vi "resave_camera_images.vi"() -> ()   [LabVIEW 2019]
uses:
  <vilib>/vision/NI_Vision_Development_Module.lvlib
panel:
  out "Processed Frames/s 8":dbl
  out "Processed Frames/s 7":dbl
  out "Processed Frames/s 6":dbl
  out "Processed Frames/s 5":dbl
  out "Processed Frames/s 4":dbl
  out "Processed Frames/s 3":dbl
  out "Processed Frames/s 2":dbl
  out "Processed Frames/s":dbl
  out "error out":errorcluster
  in  "Experiment Folder In":string="C:\\Data\\20200217_HeadTailContinuousGWN_test\\Data20200217_115033\\"
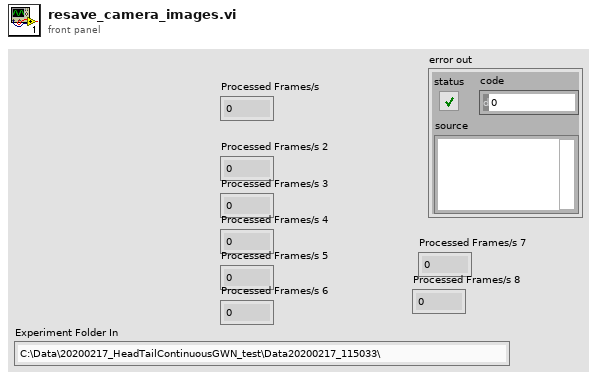
[diagram p1: front panel]
types:
  T1 = typedef "Image Type" = u32
  T2 = typedef "IMAQ Image.ctl" = refnum<image>
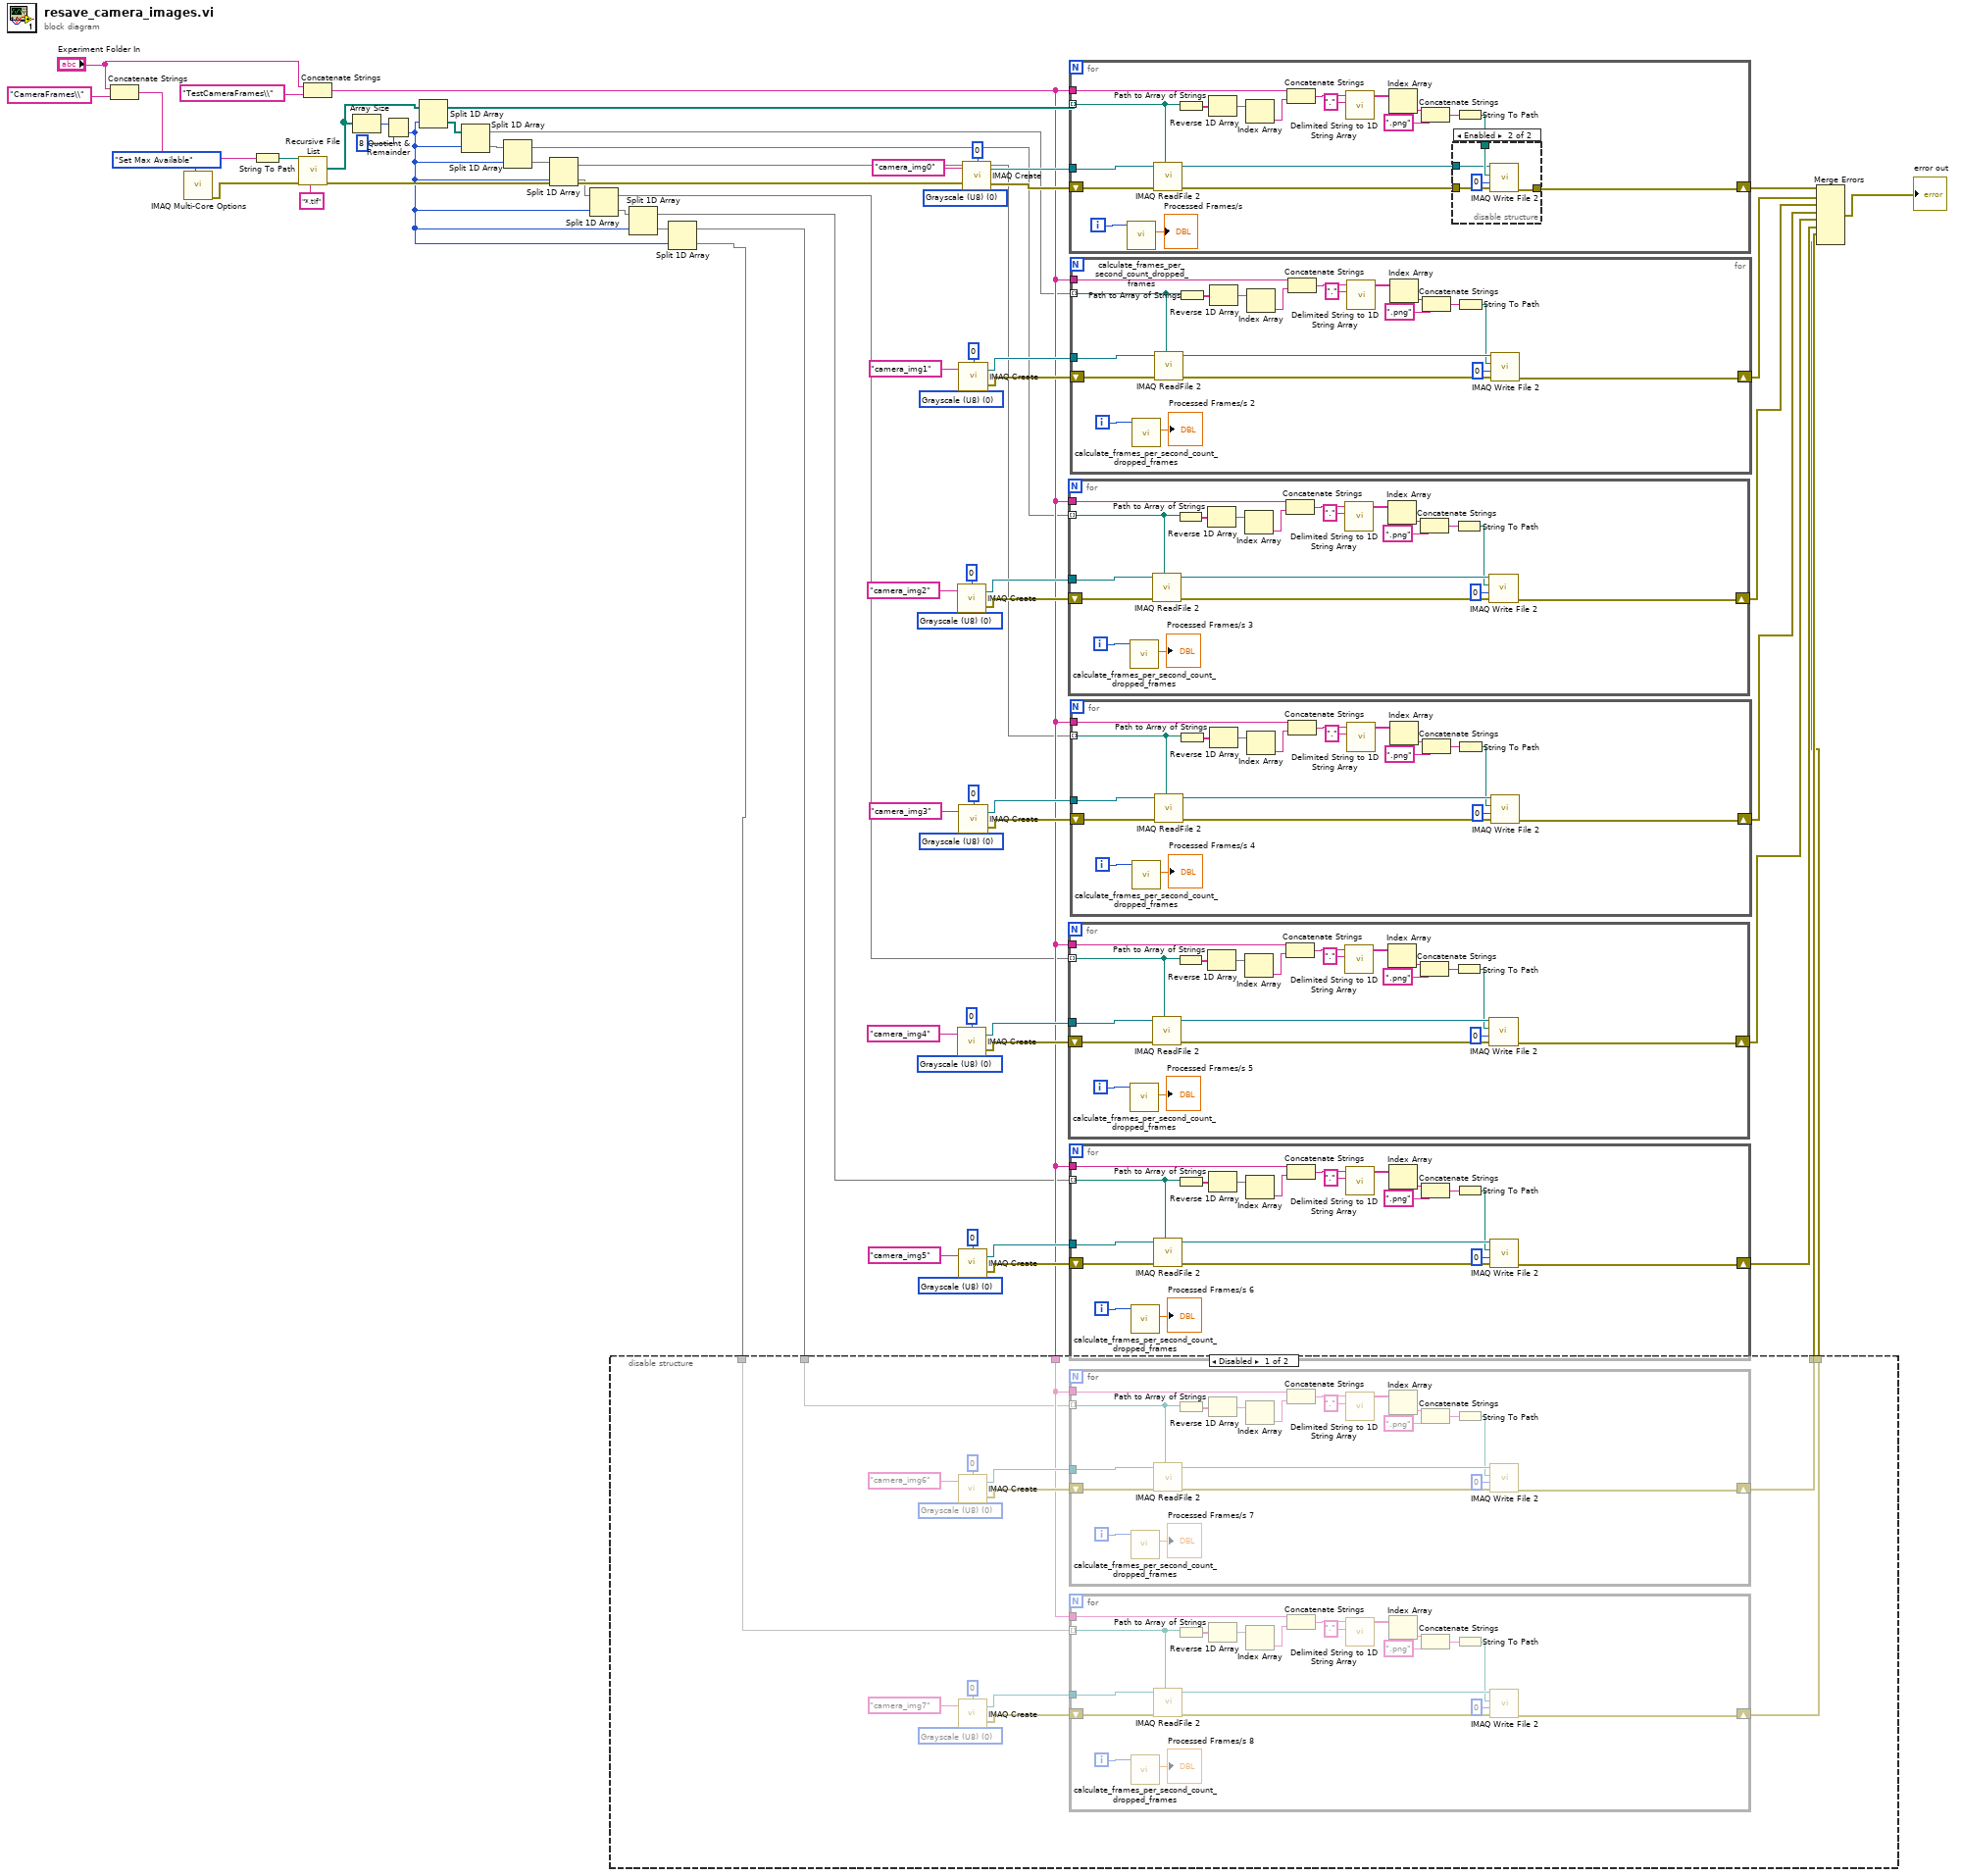
[diagram p0: block diagram]
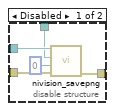
[diagram p3: hidden frame]
diagram:
  w24 = T1 0 items=["Grayscale (U8)", "Grayscale (I16)", "Grayscale (SGL)", "Complex (CSG)", "RGB (U32)", "HSL (U32)", "RGB (U64)", "Grayscale (U16)"] ("Image Type")
  w29 = T1 0 items=["Grayscale (U8)", "Grayscale (I16)", "Grayscale (SGL)", "Complex (CSG)", "RGB (U32)", "HSL (U32)", "RGB (U64)", "Grayscale (U16)"] ("Image Type")
  w34 = T1 0 items=["Grayscale (U8)", "Grayscale (I16)", "Grayscale (SGL)", "Complex (CSG)", "RGB (U32)", "HSL (U32)", "RGB (U64)", "Grayscale (U16)"] ("Image Type")
  w39 = T1 0 items=["Grayscale (U8)", "Grayscale (I16)", "Grayscale (SGL)", "Complex (CSG)", "RGB (U32)", "HSL (U32)", "RGB (U64)", "Grayscale (U16)"] ("Image Type")
  w52 = T1 0 items=["Grayscale (U8)", "Grayscale (I16)", "Grayscale (SGL)", "Complex (CSG)", "RGB (U32)", "HSL (U32)", "RGB (U64)", "Grayscale (U16)"] ("Image Type")
  w61 = T1 0 items=["Grayscale (U8)", "Grayscale (I16)", "Grayscale (SGL)", "Complex (CSG)", "RGB (U32)", "HSL (U32)", "RGB (U64)", "Grayscale (U16)"] ("Image Type")
  n1 = Concatenate Strings("Experiment Folder In", "CameraFrames\\" ("string")) -> (w66:string)
  n2 = call "IMAQ Multi-Core Options"("Get/Set Number of Cores (Get)"=enum32{"Get", "Set", "Set Max Available"}."Set Max Available") -> ("error out"=w42:errorcluster)  [unwired: 9 in, 1 out]
  n3 = String To Path(string=w66) -> (path=w64:path)
  n4 = call <vilib>:"Recursive File List.vi"("pattern"="*.tif", "error in (no error)"=w42, "Folder Path"=w64) -> ("error out"=w58:errorcluster, "All Files in Dir"=w49:path[])  [unwired: 4 in, 3 out]
  n5 = Concatenate Strings("Experiment Folder In", "TestCameraFrames\\" ("string")) -> (w21:string)
  n6 = Array Size(array=w49) -> (size(s)=w48:i32)
  n7 = Quotient & Remainder(x=w48, y=8) -> (floor(x/y)=w2:i32)  [unwired: 1 out]
  n8 = Split 1D Array(array=w49, index=w2) -> (first subarray=w55:path[], second subarray=w14:path[])
  n9 = Split 1D Array(array=w14, index=w2) -> (first subarray=w13:path[], second subarray=w12:path[])
  n10 = Split 1D Array(array=w12, index=w2) -> (first subarray=w11:path[], second subarray=w10:path[])
  n11 = Split 1D Array(array=w10, index=w2) -> (first subarray=w9:path[], second subarray=w8:path[])
  n12 = Split 1D Array(array=w8, index=w2) -> (first subarray=w7:path[], second subarray=w6:path[])
  n13 = Split 1D Array(array=w6, index=w2) -> (first subarray=w5:path[], second subarray=w4:path[])
  n14 = Split 1D Array(array=w4, index=w2) -> (first subarray=w3:path[], second subarray=w1:path[])
  n15 = disable-structure shown="Disabled" {
    disable-tunnel: w21 -> [w72 _]
    disable-tunnel: [w71 _] -> w16
    disable-tunnel: [w70 _] -> w15
    disable-tunnel: w3 -> [w69 _]
    disable-tunnel: w1 -> [w68 _]
    frame Disabled {
      w75 = T1 0 items=["Grayscale (U8)", "Grayscale (I16)", "Grayscale (SGL)", "Complex (CSG)", "RGB (U32)", "HSL (U32)", "RGB (U64)", "Grayscale (U16)"] ("Image Type")
      w80 = T1 0 items=["Grayscale (U8)", "Grayscale (I16)", "Grayscale (SGL)", "Complex (CSG)", "RGB (U32)", "HSL (U32)", "RGB (U64)", "Grayscale (U16)"] ("Image Type")
      n16 = call "IMAQ Create"("Border Size"=0, "Image Name"="camera_img6", "Image Type"=w80) -> ("New Image"=w78:T2, "error out"=w79:errorcluster)  [unwired: 2 in]
      n17 = call "IMAQ Create"("Border Size"=0, "Image Name"="camera_img7", "Image Type"=w75) -> ("New Image"=w73:T2, "error out"=w74:errorcluster)  [unwired: 2 in]
      n18 = for {
        tunnel: w69 -> [w116] mode=indexing
        tunnel: w78 -> [w122]
        tunnel: w72 -> [w115]
        shift-right: [w112] -> w71
        shift-left: w79 -> [w121]
        i -> [w111]
        n19 = call "calculate_frames_per_second_count_dropped_frames.vi"("Buffer Number"=w111) -> ("Processed Frames/s"=→"Processed Frames/s 7":dbl)  [unwired: 8 in, 2 out]
        n20 = call "IMAQ ReadFile 2"("File Path"=w116, "error in (no error)"=w121, "Image"=w122) -> ("error out"=w120:errorcluster, "Image Out"=w119:T2)  [unwired: 4 in, 3 out]
        n21 = Path to Array of Strings(0:w116) -> (2:w118:string[])  [unwired: 1 out]
        n22 = Reverse 1D Array(array=w118) -> (reversed array=w117:string[])
        n23 = Index Array(array=w117) -> (element=w114:string)  [unwired: 1 in]
        n24 = Concatenate Strings(w115, w114) -> (w109:string)
        n25 = call <vilib>:"Delimited String to 1D String Array.vi"("delimiter"=".", "delimited string"=w109) -> ("string array"=w107:string[])  [unwired: 9 in]
        n26 = Index Array(array=w107) -> (element=w106:string)  [unwired: 1 in]
        n27 = Concatenate Strings(w106, ".png" ("string")) -> (w104:string)
        n28 = String To Path(string=w104) -> (path=w113:path)
        n29 = call-poly "IMAQ Write File 2"("error in (no error)"=w120, "Image Quality"=u32 0, "File Path"=w113, "Image"=w119) -> ("error out"=w112:errorcluster)  [unwired: 6 in, 1 out]
      }
      n30 = for {
        tunnel: w68 -> [w96] mode=indexing
        tunnel: w73 -> [w102]
        tunnel: w72 -> [w95]
        shift-right: [w92] -> w70
        shift-left: w74 -> [w101]
        i -> [w91]
        n31 = call "calculate_frames_per_second_count_dropped_frames.vi"("Buffer Number"=w91) -> ("Processed Frames/s"=→"Processed Frames/s 8":dbl)  [unwired: 8 in, 2 out]
        n32 = call "IMAQ ReadFile 2"("File Path"=w96, "error in (no error)"=w101, "Image"=w102) -> ("error out"=w100:errorcluster, "Image Out"=w99:T2)  [unwired: 4 in, 3 out]
        n33 = Path to Array of Strings(0:w96) -> (2:w98:string[])  [unwired: 1 out]
        n34 = Reverse 1D Array(array=w98) -> (reversed array=w97:string[])
        n35 = Index Array(array=w97) -> (element=w94:string)  [unwired: 1 in]
        n36 = Concatenate Strings(w95, w94) -> (w89:string)
        n37 = call <vilib>:"Delimited String to 1D String Array.vi"("delimiter"=".", "delimited string"=w89) -> ("string array"=w87:string[])  [unwired: 9 in]
        n38 = Index Array(array=w87) -> (element=w86:string)  [unwired: 1 in]
        n39 = Concatenate Strings(w86, ".png" ("string")) -> (w84:string)
        n40 = String To Path(string=w84) -> (path=w93:path)
        n41 = call-poly "IMAQ Write File 2"("error in (no error)"=w100, "Image Quality"=u32 0, "File Path"=w93, "Image"=w99) -> ("error out"=w92:errorcluster)  [unwired: 6 in, 1 out]
      }
    }
    frame Enabled {
    }
  }
  n42 = call "IMAQ Create"("Border Size"=0, "Image Name"="camera_img2", "Image Type"=w39) -> ("New Image"=w37:T2, "error out"=w38:errorcluster)  [unwired: 2 in]
  n43 = call "IMAQ Create"("Border Size"=0, "Image Name"="camera_img4", "Image Type"=w29) -> ("New Image"=w27:T2, "error out"=w28:errorcluster)  [unwired: 2 in]
  n44 = call "IMAQ Create"("Border Size"=0, "Image Name"="camera_img5", "Image Type"=w24) -> ("New Image"=w22:T2, "error out"=w23:errorcluster)  [unwired: 2 in]
  n45 = call "IMAQ Create"("Border Size"=0, "Image Name"="camera_img1", "Image Type"=w52) -> ("New Image"=w50:T2, "error out"=w51:errorcluster)  [unwired: 2 in]
  n46 = call "IMAQ Create"("Border Size"=0, "Image Name"="camera_img3", "Image Type"=w34) -> ("New Image"=w32:T2, "error out"=w33:errorcluster)  [unwired: 2 in]
  n47 = call "IMAQ Create"("Border Size"=0, "Image Name"="camera_img0", "Image Type"=w61, "error in (no error)"=w58) -> ("New Image"=w60:T2, "error out"=w59:errorcluster)  [unwired: 1 in]
  n48 = for {
    tunnel: w11 -> [w136] mode=indexing
    tunnel: w37 -> [w142]
    tunnel: w21 -> [w135]
    shift-right: [w132] -> w20
    shift-left: w38 -> [w141]
    i -> [w131]
    n49 = call "calculate_frames_per_second_count_dropped_frames.vi"("Buffer Number"=w131) -> ("Processed Frames/s"=→"Processed Frames/s 3":dbl)  [unwired: 8 in, 2 out]
    n50 = call "IMAQ ReadFile 2"("File Path"=w136, "error in (no error)"=w141, "Image"=w142) -> ("error out"=w140:errorcluster, "Image Out"=w139:T2)  [unwired: 4 in, 3 out]
    n51 = Path to Array of Strings(0:w136) -> (2:w138:string[])  [unwired: 1 out]
    n52 = Reverse 1D Array(array=w138) -> (reversed array=w137:string[])
    n53 = Index Array(array=w137) -> (element=w134:string)  [unwired: 1 in]
    n54 = Concatenate Strings(w135, w134) -> (w129:string)
    n55 = call <vilib>:"Delimited String to 1D String Array.vi"("delimiter"=".", "delimited string"=w129) -> ("string array"=w127:string[])  [unwired: 9 in]
    n56 = Index Array(array=w127) -> (element=w126:string)  [unwired: 1 in]
    n57 = Concatenate Strings(w126, ".png" ("string")) -> (w124:string)
    n58 = String To Path(string=w124) -> (path=w133:path)
    n59 = call-poly "IMAQ Write File 2"("error in (no error)"=w140, "Image Quality"=u32 0, "File Path"=w133, "Image"=w139) -> ("error out"=w132:errorcluster)  [unwired: 6 in, 1 out]
  }
  n60 = for {
    tunnel: w7 -> [w156] mode=indexing
    tunnel: w27 -> [w162]
    tunnel: w21 -> [w155]
    shift-right: [w152] -> w18
    shift-left: w28 -> [w161]
    i -> [w151]
    n61 = call "calculate_frames_per_second_count_dropped_frames.vi"("Buffer Number"=w151) -> ("Processed Frames/s"=→"Processed Frames/s 5":dbl)  [unwired: 8 in, 2 out]
    n62 = call "IMAQ ReadFile 2"("File Path"=w156, "error in (no error)"=w161, "Image"=w162) -> ("error out"=w160:errorcluster, "Image Out"=w159:T2)  [unwired: 4 in, 3 out]
    n63 = Path to Array of Strings(0:w156) -> (2:w158:string[])  [unwired: 1 out]
    n64 = Reverse 1D Array(array=w158) -> (reversed array=w157:string[])
    n65 = Index Array(array=w157) -> (element=w154:string)  [unwired: 1 in]
    n66 = Concatenate Strings(w155, w154) -> (w149:string)
    n67 = call <vilib>:"Delimited String to 1D String Array.vi"("delimiter"=".", "delimited string"=w149) -> ("string array"=w147:string[])  [unwired: 9 in]
    n68 = Index Array(array=w147) -> (element=w146:string)  [unwired: 1 in]
    n69 = Concatenate Strings(w146, ".png" ("string")) -> (w144:string)
    n70 = String To Path(string=w144) -> (path=w153:path)
    n71 = call-poly "IMAQ Write File 2"("error in (no error)"=w160, "Image Quality"=u32 0, "File Path"=w153, "Image"=w159) -> ("error out"=w152:errorcluster)  [unwired: 6 in, 1 out]
  }
  n72 = for {
    tunnel: w55 -> [w175] mode=indexing
    tunnel: w60 -> [w181]
    tunnel: w21 -> [w174]
    shift-right: [w171] -> w46
    shift-left: w59 -> [w180]
    i -> [w170]
    n73 = call "calculate_frames_per_second_count_dropped_frames.vi"("Buffer Number"=w170) -> ("Processed Frames/s"=→"Processed Frames/s":dbl)  [unwired: 8 in, 2 out]
    n74 = call "IMAQ ReadFile 2"("File Path"=w175, "error in (no error)"=w180, "Image"=w181) -> ("error out"=w179:errorcluster, "Image Out"=w178:T2)  [unwired: 4 in, 3 out]
    n75 = Path to Array of Strings(0:w175) -> (2:w177:string[])  [unwired: 1 out]
    n76 = Reverse 1D Array(array=w177) -> (reversed array=w176:string[])
    n77 = Index Array(array=w176) -> (element=w173:string)  [unwired: 1 in]
    n78 = Concatenate Strings(w174, w173) -> (w168:string)
    n79 = call <vilib>:"Delimited String to 1D String Array.vi"("delimiter"=".", "delimited string"=w168) -> ("string array"=w166:string[])  [unwired: 9 in]
    n80 = Index Array(array=w166) -> (element=w165:string)  [unwired: 1 in]
    n81 = Concatenate Strings(w165, ".png" ("string")) -> (w163:string)
    n82 = String To Path(string=w163) -> (path=w172:path)
    n83 = disable-structure shown="Enabled" {
      disable-tunnel: w179 -> [w186 w191]
      disable-tunnel: w178 -> [w185 w188]
      disable-tunnel: w172 -> [w184 w189]
      disable-tunnel: [w183 w190] -> w171
      frame Disabled {
        n84 = call "nivision_savepng.vi"("error in (no error)"=w186, "Image Quality"=u32 0, "File Path"=w184, "Image"=w185) -> ("error out"=w183:errorcluster)  [unwired: 6 in, 1 out]
      }
      frame Enabled {
        n85 = call-poly "IMAQ Write File 2"("error in (no error)"=w191, "Image Quality"=u32 0, "File Path"=w189, "Image"=w188) -> ("error out"=w190:errorcluster)  [unwired: 6 in, 1 out]
      }
    }
  }
  n86 = for {
    tunnel: w5 -> [w205] mode=indexing
    tunnel: w22 -> [w211]
    tunnel: w21 -> [w204]
    shift-right: [w201] -> w17
    shift-left: w23 -> [w210]
    i -> [w200]
    n87 = call "calculate_frames_per_second_count_dropped_frames.vi"("Buffer Number"=w200) -> ("Processed Frames/s"=→"Processed Frames/s 6":dbl)  [unwired: 8 in, 2 out]
    n88 = call "IMAQ ReadFile 2"("File Path"=w205, "error in (no error)"=w210, "Image"=w211) -> ("error out"=w209:errorcluster, "Image Out"=w208:T2)  [unwired: 4 in, 3 out]
    n89 = Path to Array of Strings(0:w205) -> (2:w207:string[])  [unwired: 1 out]
    n90 = Reverse 1D Array(array=w207) -> (reversed array=w206:string[])
    n91 = Index Array(array=w206) -> (element=w203:string)  [unwired: 1 in]
    n92 = Concatenate Strings(w204, w203) -> (w198:string)
    n93 = call <vilib>:"Delimited String to 1D String Array.vi"("delimiter"=".", "delimited string"=w198) -> ("string array"=w196:string[])  [unwired: 9 in]
    n94 = Index Array(array=w196) -> (element=w195:string)  [unwired: 1 in]
    n95 = Concatenate Strings(w195, ".png" ("string")) -> (w193:string)
    n96 = String To Path(string=w193) -> (path=w202:path)
    n97 = call-poly "IMAQ Write File 2"("error in (no error)"=w209, "Image Quality"=u32 0, "File Path"=w202, "Image"=w208) -> ("error out"=w201:errorcluster)  [unwired: 6 in, 1 out]
  }
  n98 = for {
    tunnel: w13 -> [w225] mode=indexing
    tunnel: w50 -> [w231]
    tunnel: w21 -> [w224]
    shift-right: [w221] -> w44
    shift-left: w51 -> [w230]
    i -> [w220]
    n99 = call "calculate_frames_per_second_count_dropped_frames.vi"("Buffer Number"=w220) -> ("Processed Frames/s"=→"Processed Frames/s 2":dbl)  [unwired: 8 in, 2 out]
    n100 = call "IMAQ ReadFile 2"("File Path"=w225, "error in (no error)"=w230, "Image"=w231) -> ("error out"=w229:errorcluster, "Image Out"=w228:T2)  [unwired: 4 in, 3 out]
    n101 = Path to Array of Strings(0:w225) -> (2:w227:string[])  [unwired: 1 out]
    n102 = Reverse 1D Array(array=w227) -> (reversed array=w226:string[])
    n103 = Index Array(array=w226) -> (element=w223:string)  [unwired: 1 in]
    n104 = Concatenate Strings(w224, w223) -> (w218:string)
    n105 = call <vilib>:"Delimited String to 1D String Array.vi"("delimiter"=".", "delimited string"=w218) -> ("string array"=w216:string[])  [unwired: 9 in]
    n106 = Index Array(array=w216) -> (element=w215:string)  [unwired: 1 in]
    n107 = Concatenate Strings(w215, ".png" ("string")) -> (w213:string)
    n108 = String To Path(string=w213) -> (path=w222:path)
    n109 = call-poly "IMAQ Write File 2"("error in (no error)"=w229, "Image Quality"=u32 0, "File Path"=w222, "Image"=w228) -> ("error out"=w221:errorcluster)  [unwired: 6 in, 1 out]
  }
  n110 = for {
    tunnel: w9 -> [w245] mode=indexing
    tunnel: w32 -> [w251]
    tunnel: w21 -> [w244]
    shift-right: [w241] -> w19
    shift-left: w33 -> [w250]
    i -> [w240]
    n111 = call "calculate_frames_per_second_count_dropped_frames.vi"("Buffer Number"=w240) -> ("Processed Frames/s"=→"Processed Frames/s 4":dbl)  [unwired: 8 in, 2 out]
    n112 = call "IMAQ ReadFile 2"("File Path"=w245, "error in (no error)"=w250, "Image"=w251) -> ("error out"=w249:errorcluster, "Image Out"=w248:T2)  [unwired: 4 in, 3 out]
    n113 = Path to Array of Strings(0:w245) -> (2:w247:string[])  [unwired: 1 out]
    n114 = Reverse 1D Array(array=w247) -> (reversed array=w246:string[])
    n115 = Index Array(array=w246) -> (element=w243:string)  [unwired: 1 in]
    n116 = Concatenate Strings(w244, w243) -> (w238:string)
    n117 = call <vilib>:"Delimited String to 1D String Array.vi"("delimiter"=".", "delimited string"=w238) -> ("string array"=w236:string[])  [unwired: 9 in]
    n118 = Index Array(array=w236) -> (element=w235:string)  [unwired: 1 in]
    n119 = Concatenate Strings(w235, ".png" ("string")) -> (w233:string)
    n120 = String To Path(string=w233) -> (path=w242:path)
    n121 = call-poly "IMAQ Write File 2"("error in (no error)"=w249, "Image Quality"=u32 0, "File Path"=w242, "Image"=w248) -> ("error out"=w241:errorcluster)  [unwired: 6 in, 1 out]
  }
  n122 = Merge Errors(w46, w44, w20, w19, w18, w17, w16, w15) -> (→"error out":errorcluster)
